vi "DCHX Dehumidification Setup_V17.vi"() -> ()   [LabVIEW 2018]
uses:
  <vilib>/DAQmx/write.llb/DAQmx Write (Analog DBL 1Chan 1Samp).vi
  <vilib>/DAQmx/write.llb/DAQmx Write (Digital Bool 1Line 1Point).vi
  <vilib>/DAQmx/read.llb/DAQmx Read (Analog 1D Wfm NChan 1Samp).vi
  <vilib>/DAQmx/create/channels.llb/DAQmx Create Channel (AI-Temperature-Thermocouple).vi
  <vilib>/DAQmx/create/channels.llb/DAQmx Create Channel (AI-Voltage-Basic).vi
  <vilib>/DAQmx/create/channels.llb/DAQmx Create Channel (DO-Digital Output).vi
  <vilib>/Instr/_visa.llb/VISA Configure Serial Port (Instr).vi
  <vilib>/DAQmx/create/channels.llb/DAQmx Create Channel (AO-Voltage-Basic).vi
  <vilib>/DAQmx/create/channels.llb/DAQmx Create Channel (AI-Current-Basic).vi
  <vilib>/DAQmx/miscellaneous.llb/DAQmx Fill In Error Info.vi
  <vilib>/Waveform/WDTOps.llb/WDT Get XY Value DBL.vi
  <vilib>/Analysis/polynomials.llb/Scalar Polynomial Evaluation (DBL).vi
  <resource>/objmgr/daqmx.rc
  <vilib>/Analysis/NI_AALPro.lvlib
panel:
  in  "Reset":bool
  out "RH2":dbl
  out "RH1":dbl
  out "error out 3":errorcluster
  out "error out 2":errorcluster
  in  "Tab Control 1":enum32{"Controls", "Channels", "Calibration"}(tab)
  in  "Cold Chiller Power":bool
  in  "Cold Chiller Setpoint":dbl=30.0 format="%.3g"
  in  "Hot Chiller Power":bool
  in  "Hot Chiller Setpoint":dbl=30.0 format="%.3g"
  in  "Fan Speed Setpoint (0-10V)":dbl min=0.0 max=10.0
  in  "Start test":bool
  in  "Number of complete cycles":dbl
  out "Number of Half-Cycles":dbl
  in  "Heating time (sec)":dbl=7.0 caption="Time Target (s)"
  in  "Cooling time (sec)":dbl=3.0 caption="Time Target (s)"
  out "Elapsed Half-Cycle Time (s)":dbl format="%#_3g"
  in  "Heating/Cooling Status":bool
  in  "Humidity/Temp Sensors":tag="cDAQ6Mod1/ai0:3"
  in  "Thermocouples":tag="cDAQ6Mod2/ai0:1"
  in  "Solenoid Channel":tag="cDAQ6Mod4/port0/line0"
  in  "Solenoid Channel 2":tag="cDAQ6Mod4/port0/line1"
  in  "Cold Chiller Port":refnum<visa-resource-name>="COM3"
  in  "Hot Chiller Port":refnum<visa-resource-name>="COM3"
  in  "Fans (Output)":tag="cDAQ6Mod3/ao0"
  in  "DUK Flow Meter":tag="cDAQ6Mod1/ai9"
  in  "Differential Pressure Current":tag="cDAQ6Mod1/ai8"
  in  "DUK FLow Meter scale":dbl=1245.0 format="%0.2f"
  in  "DUK FLow Meter offset":dbl=-4.9
  in  "RTD1 offset":dbl=-2.53 format="%0.2f"
  in  "RTD2 offset":dbl=-3.22 format="%0.2f"
  in  "RTD1 scale":dbl=5.6286 format="%0.2f"
  in  "RTD2 scale":dbl=5.701 format="%0.2f"
  in  "RH1 offset":ext=0.1906
  in  "RH2 offset":ext=0.246
  in  "RH1  scale":ext=10.58
  in  "RH2 scale":ext=10.3599999999999999997
  in  "TC-T1 offset":dbl format="%0.2f"
  in  "TC-T1 scale":dbl=1.0 format="%0.2f"
  in  "TC-T2 offset":dbl format="%0.2f"
  in  "TC-T2 scale":dbl=1.0 format="%0.2f"
  in  "Scale DiffP 1":dbl=124945.0 format="%#_13g"
  in  "offset DiffP":dbl=-1504.3 format="%0.2f"
  in  "stop":bool
  in  "Tab Control 2":enum32{"All Data Graphs"}(tab)
  out "Air Flow Rate (CFM)":waveform(dbl)(graph)
  out "DUK Flow Meter":waveform(dbl)(graph)
  out "RTD Temeprature - KIMO":waveform(dbl)[](graph)
  out "Relative Humidity - KIMO":waveform(dbl)[](graph)
  out "Temperature-TC":waveform(dbl)[](graph)
  out "Absolute Humidity Chart":waveform(dbl)[](graph)
  out "Orifice Pressure (Pa)":waveform(dbl)(graph)
  out "Percent Error":dbl
  # "Cooling"
  # "Heating"
  # "Air Side"
  # "Liquid Side"
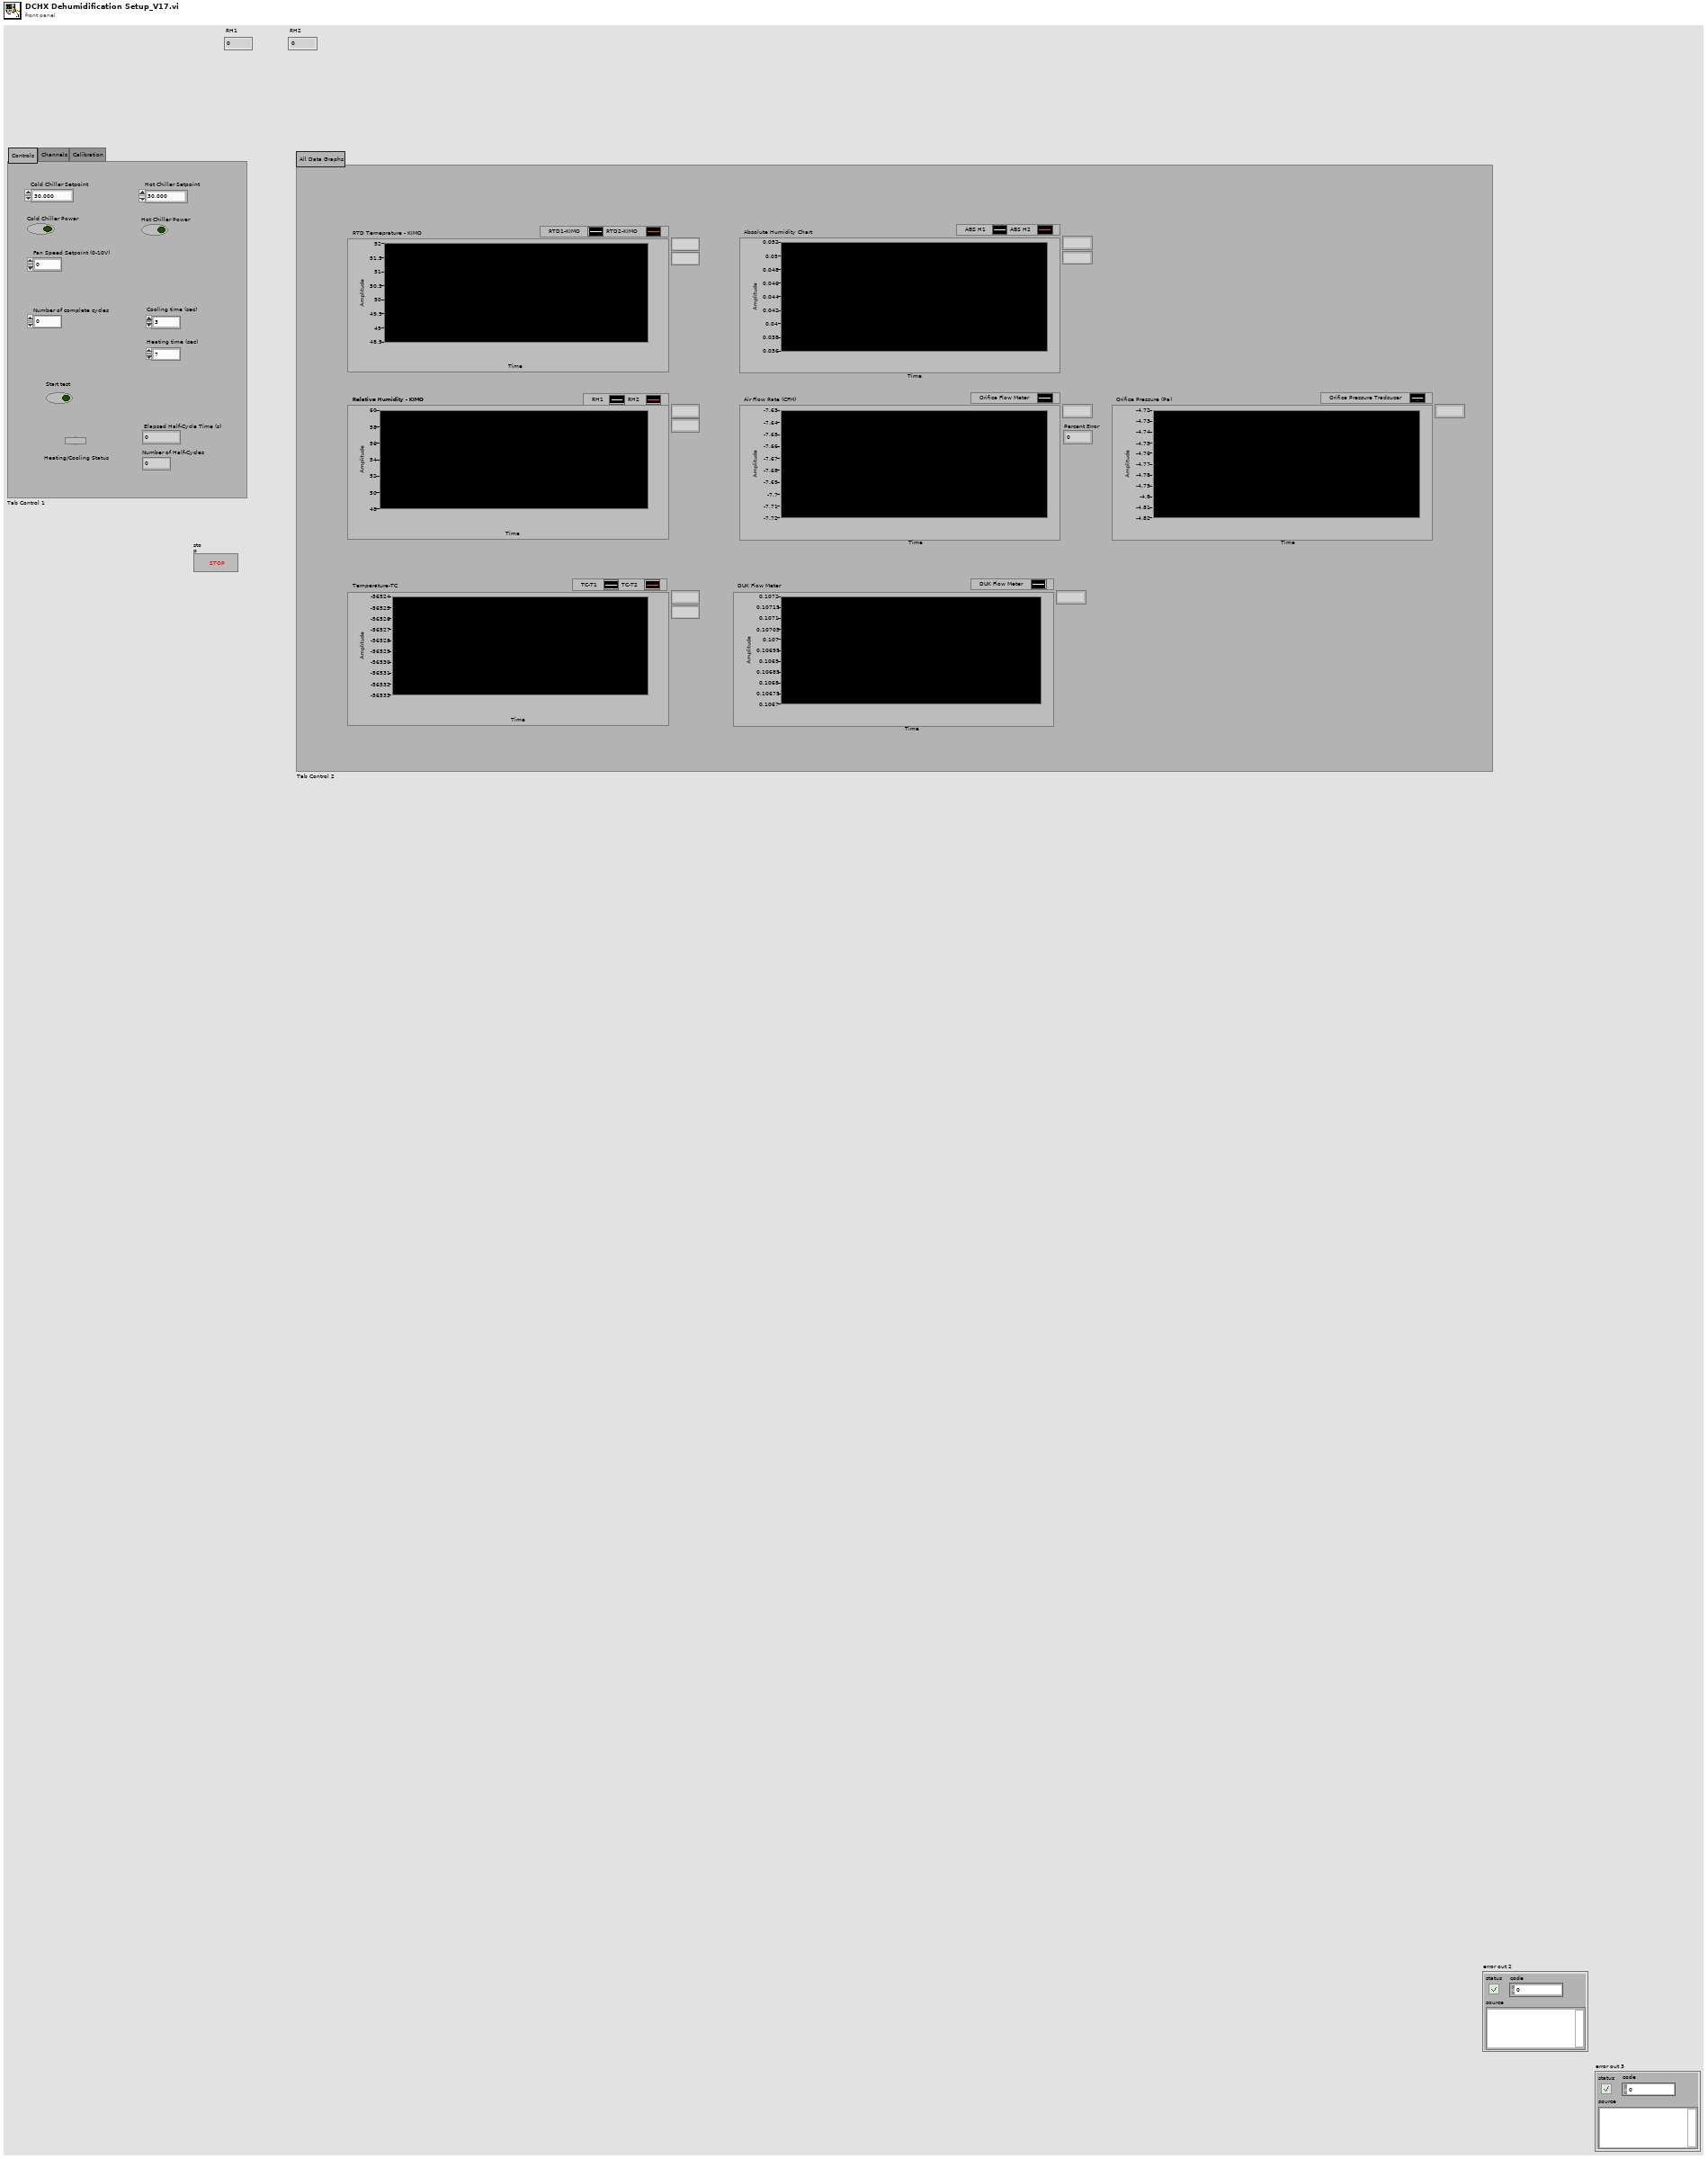
[diagram p1: front panel]
types:
  T1 = enum8{"Enabled", "Disabled", "Disabled and Grayed Out"}
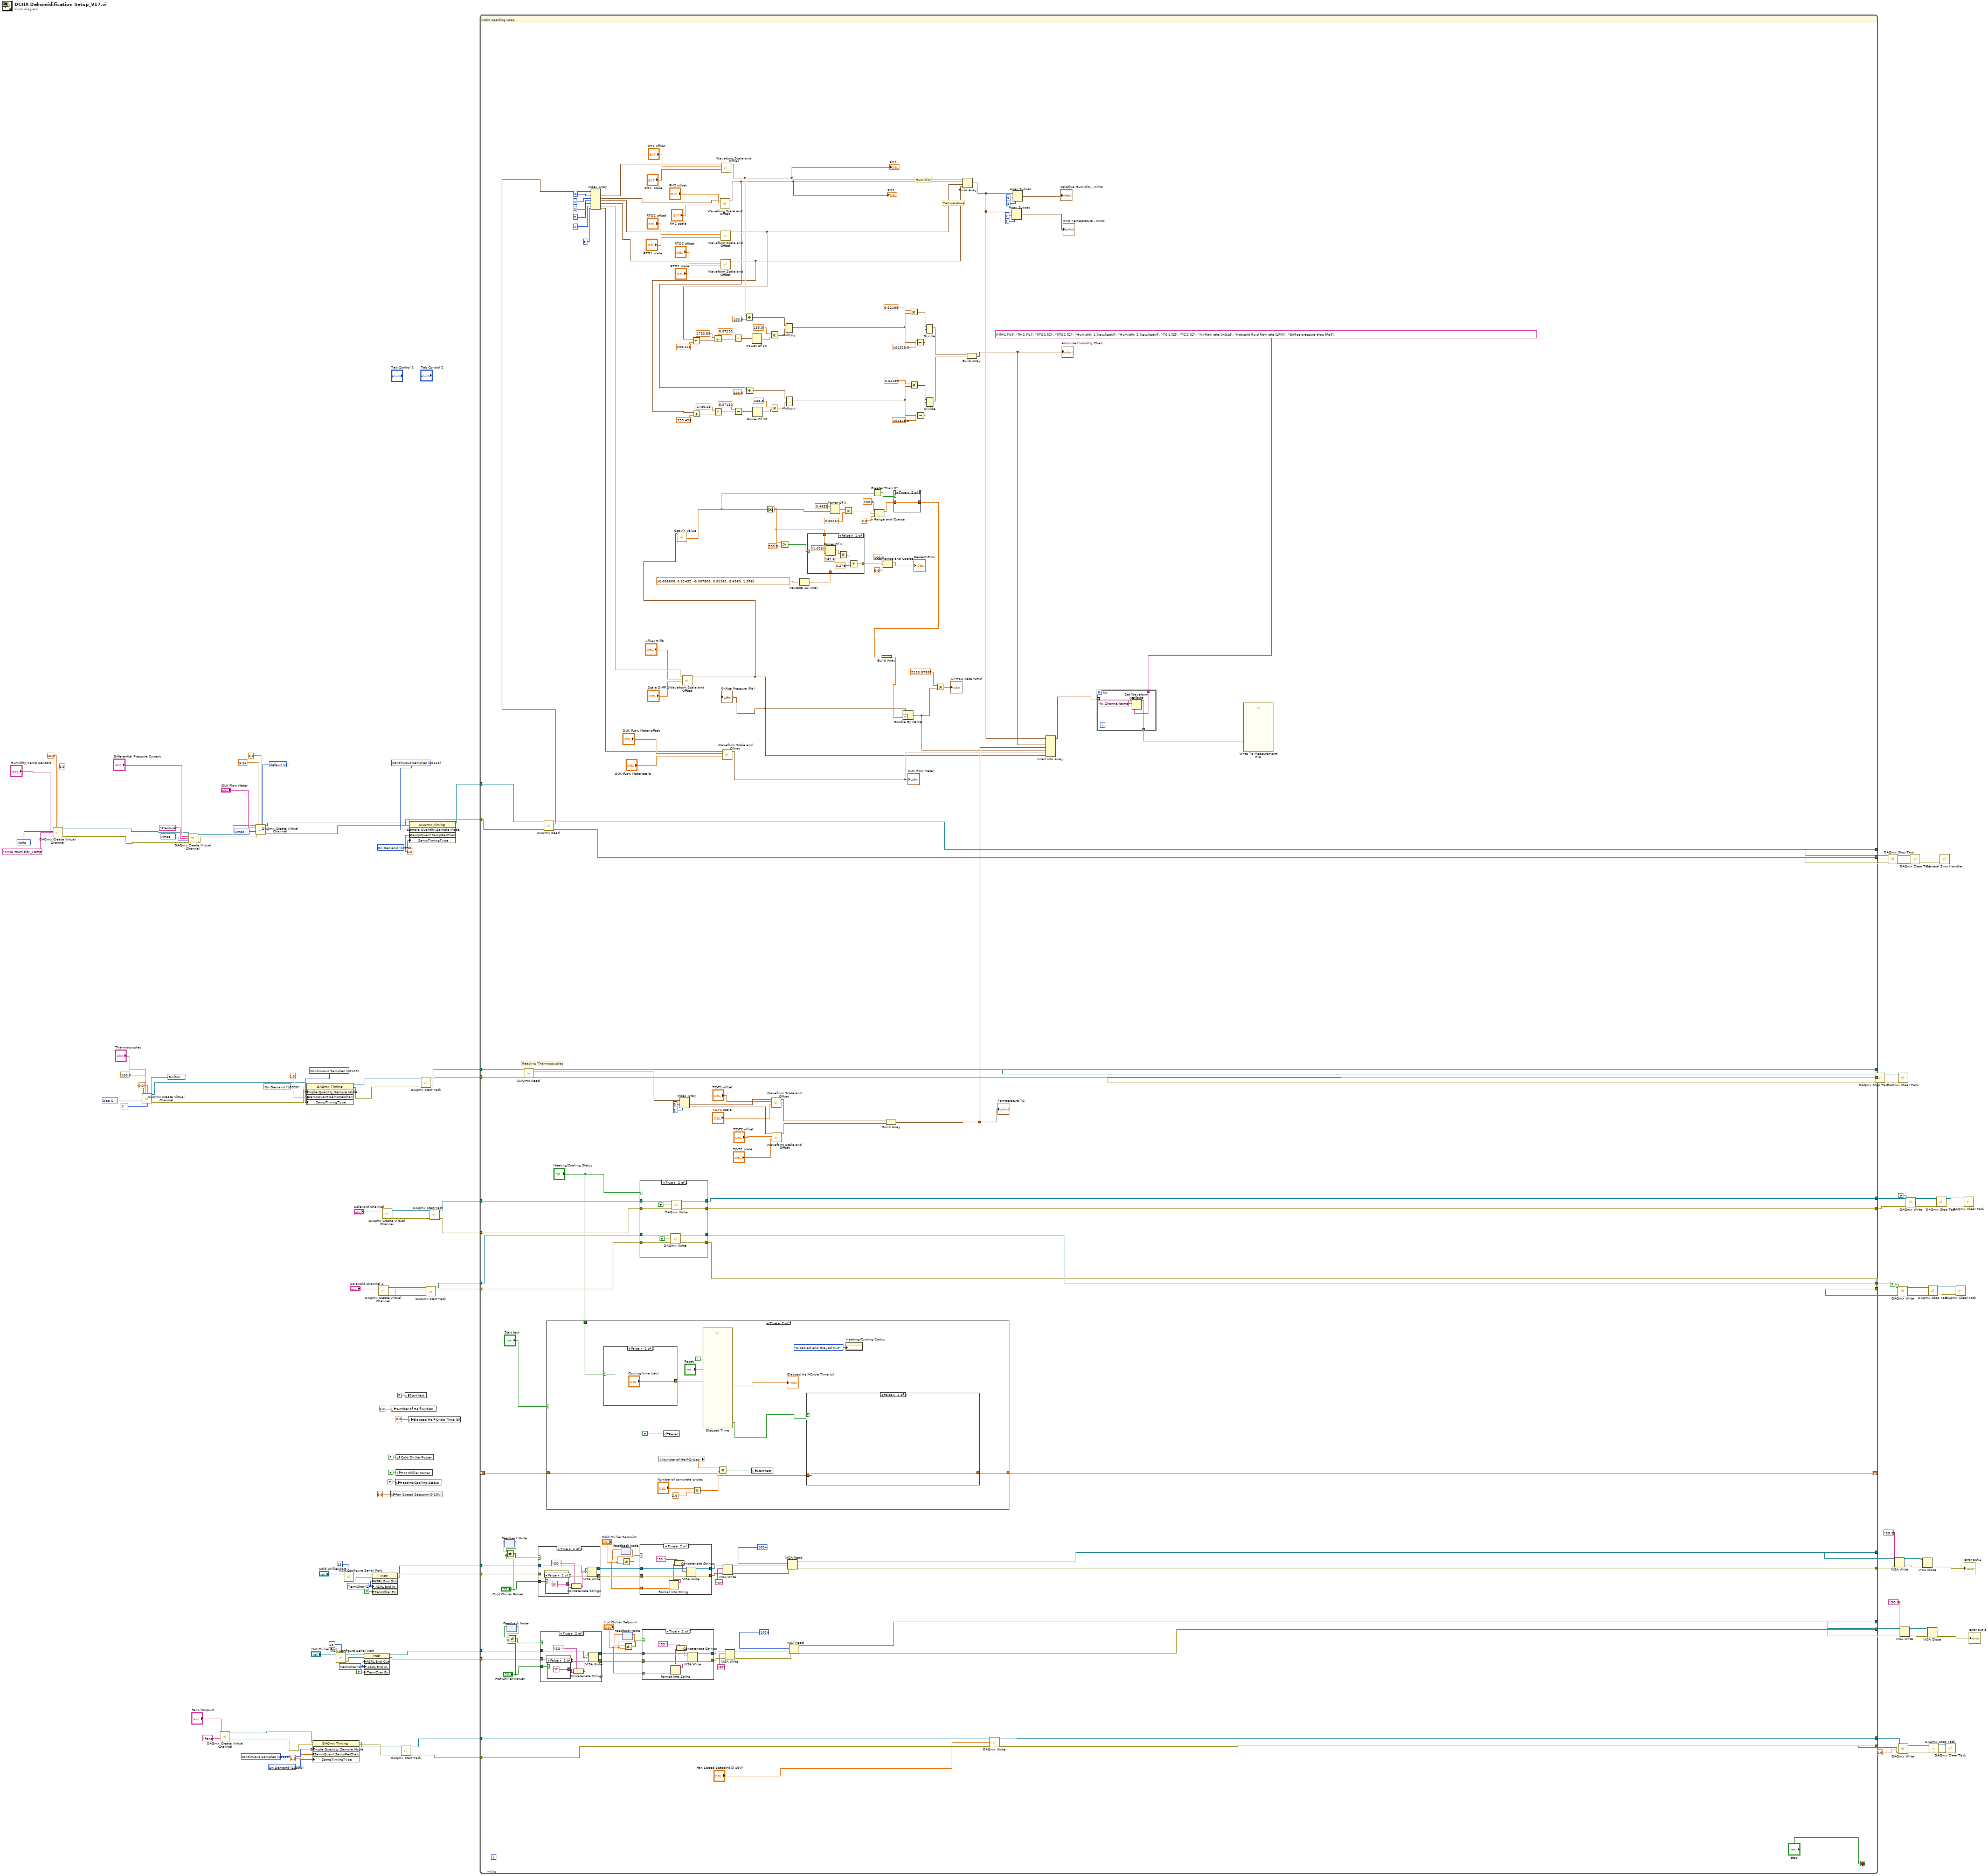
[diagram p0: block diagram]
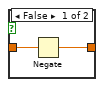
[diagram p2: hidden frame]
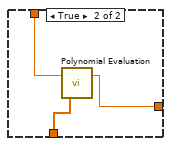
[diagram p3: hidden frame]
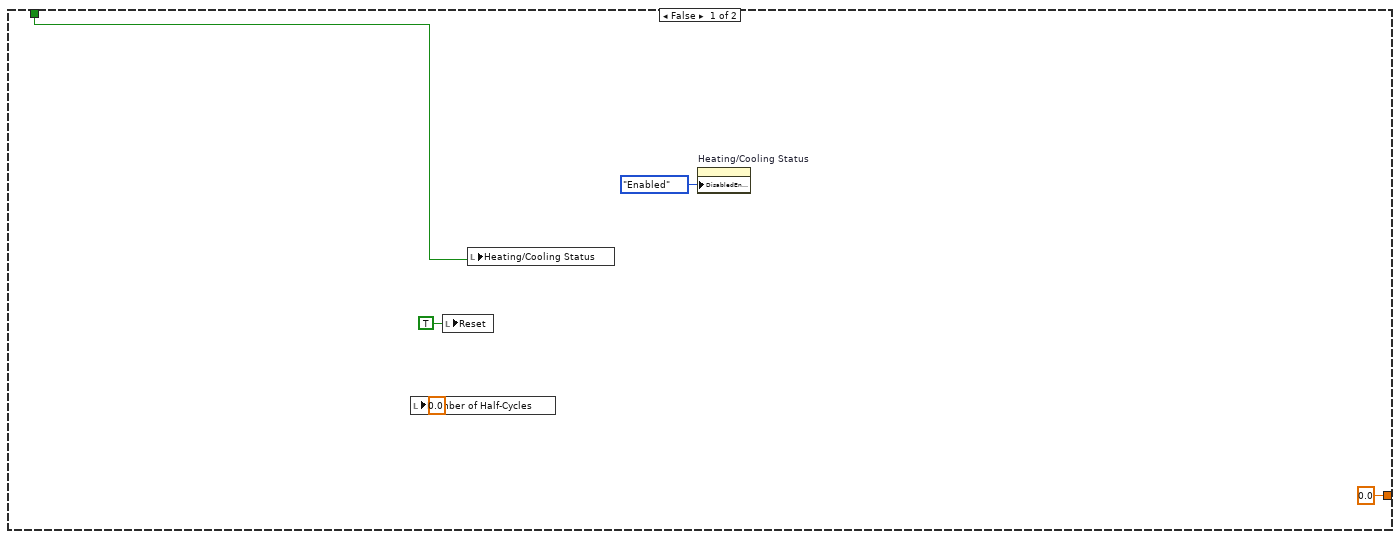
[diagram p4: hidden frame]
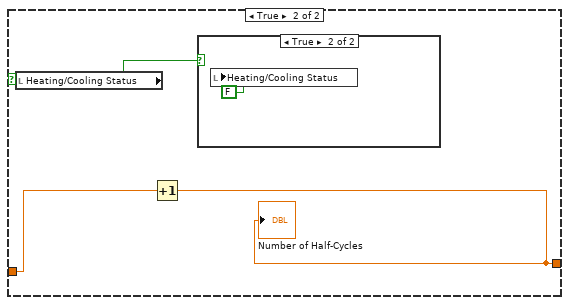
[diagram p5: hidden frame]
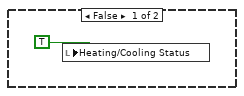
[diagram p6: hidden frame]
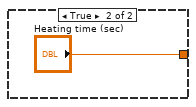
[diagram p7: hidden frame]
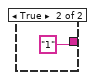
[diagram p10: hidden frame]
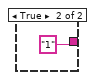
[diagram p13: hidden frame]
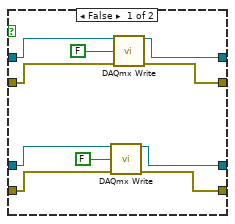
[diagram p14: hidden frame]
diagram:
  w18 = 10342 items=["Amps"=10342, "From Custom Scale"=10065] ("units")
  w23 = -1 items=["default"=-1, "RSE"=10083, "NRSE"=10078, "Differential"=10106, "Pseudodifferential"=12529] ("input terminal configuration")
  w26 = 10342 items=["Amps"=10342, "From Custom Scale"=10065] ("units")
  w38 = 10390 items=["Sample Clock"=10388, "Burst Handshake"=12548, "Handshake"=10389, "Implicit"=10451, "On Demand"=10390, "Change Detection"=12504, "Pipelined Sample Clock"=14668] ("SampTimingType")
  w40 = 10123 items=["Finite Samples"=10178, "Continuous Samples"=10123, "Hardware Timed Single Point"=12522] ("SampQuant.SampMode")
  w49 = u16 2 items=["None", "Last Bit", "TermChar"] ("Serial Settings:End Mode for Reads")
  w63 = u16 2 items=["None", "Last Bit", "TermChar"] ("Serial Settings:End Mode for Reads")
  w104 = 10348 items=["Volts"=10348, "From Custom Scale"=10065] ("units")
  w105 = 10390 items=["Sample Clock"=10388, "Burst Handshake"=12548, "Handshake"=10389, "Implicit"=10451, "On Demand"=10390, "Change Detection"=12504, "Pipelined Sample Clock"=14668] ("SampTimingType")
  w107 = 10123 items=["Finite Samples"=10178, "Continuous Samples"=10123, "Hardware Timed Single Point"=12522] ("SampQuant.SampMode")
  w112 = 10390 items=["Sample Clock"=10388, "Burst Handshake"=12548, "Handshake"=10389, "Implicit"=10451, "On Demand"=10390, "Change Detection"=12504, "Pipelined Sample Clock"=14668] ("SampTimingType")
  w113 = 10123 items=["Finite Samples"=10178, "Continuous Samples"=10123, "Hardware Timed Single Point"=12522] ("SampQuant.SampMode")
  w117 = 10086 items=["J"=10072, "K"=10073, "N"=10077, "R"=10082, "S"=10085, "T"=10086, "B"=10047, "E"=10055] ("thermocouple type")
  w118 = 10200 items=["Built-In"=10200, "Constant Value"=10116, "Channel"=10113] ("cjc source")
  w119 = 10143 items=["Deg C"=10143, "Deg F"=10144, "Kelvins"=10325, "Deg R"=10145, "From Custom Scale"=10065] ("units")
  n1 = call-poly <vilib>:"DAQmx Create Virtual Channel.vi"("maximum value"=10.0, "minimum value"=0.0, "physical channels"="Humidity/Temp Sensors", "name to assign"="KIMO Humidity_Temp", "units"=w104) -> ("task out"=w14:refnum<k21>, "error out"=w15:errorcluster)  [unwired: 9 in]
  n2 = call-poly <vilib>:"DAQmx Create Virtual Channel.vi"("maximum value"=100.0, "minimum value"=0.0, "physical channels"="Thermocouples", "cjc source"=w118, "units"=w119, "thermocouple type"=w117) -> ("task out"=w109:refnum<k21>, "error out"=w108:errorcluster)  [unwired: 8 in]
  n3 = call-poly <vilib>:"DAQmx Create Virtual Channel.vi"("task in"=w14, "physical channels"="Differential Pressure Current", "name to assign"="Pressure", "units"=w18, "error in"=w15) -> ("task out"=w17:refnum<k21>, "error out"=w16:errorcluster)  [unwired: 9 in]
  n4 = call-poly <vilib>:"DAQmx Create Virtual Channel.vi"("physical channels"="Fans (Output)", "name to assign"="Fans") -> ("task out"=w35:refnum<k21>, "error out"=w36:errorcluster)  [unwired: 12 in]
  n5 = call-poly <vilib>:"DAQmx Create Virtual Channel.vi"("task in"=w17, "maximum value"=0.02, "minimum value"=0.0, "input terminal configuration"=w23, "physical channels"="DUK Flow Meter", "units"=w26, "error in"=w16) -> ("task out"=w22:refnum<k21>, "error out"=w21:errorcluster)  [unwired: 7 in]
  n6 = property class="DAQmx Timing"(reference=w109, error in=w108, "Sample Quantity:Sample Mode"=w113, "SampQuant.SampPerChan"=1.0, "SampTimingType"=w112) -> (reference out=w111:refnum<k21>, error out=w110:errorcluster)
  n7 = property class="DAQmx Timing"(reference=w35, error in=w36, "Sample Quantity:Sample Mode"=w40, "SampQuant.SampPerChan"=1.0, "SampTimingType"=w38) -> (reference out=w29:refnum<k21>, error out=w28:errorcluster)
  n8 = call-poly "VISA Configure Serial Port"("VISA resource name"="Hot Chiller Port", "termination char\n(0xA = '\\n' = LF)"=u8 13 ("termination char\n(0xA = '\\n' = LF)")) -> ("VISA resource name out"=w46:refnum<visa-resource-name>, "error out"=w47:errorcluster)  [unwired: 12 in]
  n9 = call-poly "VISA Configure Serial Port"("VISA resource name"="Cold Chiller Port", "termination char\n(0xA = '\\n' = LF)"=u8 13 ("termination char\n(0xA = '\\n' = LF)")) -> ("VISA resource name out"=w60:refnum<visa-resource-name>, "error out"=w61:errorcluster)  [unwired: 12 in]
  n10 = property class="Instr"(reference=w46, error in=w47, "ASRL End Out"=w49, "ASRL End In"=w49, "TermChar En"=FALSE ("Message Based Settings:Termination Character Enable")) -> (reference out=w44:refnum<visa-resource-name>, error out=w43:errorcluster)
  n11 = property class="Instr"(reference=w60, error in=w61, "ASRL End Out"=w63, "ASRL End In"=w63, "TermChar En"=FALSE ("Message Based Settings:Termination Character Enable")) -> (reference out=w58:refnum<visa-resource-name>, error out=w57:errorcluster)
  n12 = call-poly <vilib>:"DAQmx Create Virtual Channel.vi"("lines"="Solenoid Channel 2") -> ("task out"=w78:refnum<k21>, "error out"=w79:errorcluster)  [unwired: 13 in]
  n13 = call-poly <vilib>:"DAQmx Create Virtual Channel.vi"("lines"="Solenoid Channel") -> ("task out"=w90:refnum<k21>, "error out"=w91:errorcluster)  [unwired: 13 in]
  n14 = local write "Fan Speed Setpoint (0-10V)"(0.0 ("Fan Speed Setpoint (0-3600 RPM)")) -> ()
  n15 = local write "Number of Half-Cycles"(0.0 ("Cycles")) -> ()
  n16 = local write "Heating/Cooling Status"(FALSE ("Heating/Cooling Status")) -> ()
  n17 = local write "Cold Chiller Power"(FALSE ("Cold Chiller Power")) -> ()
  n18 = local write "Hot Chiller Power"(FALSE ("Hot Chiller Power")) -> ()
  n19 = call <vilib>:"DAQmx Start Task.vi"("task/channels in"=w29, "error in"=w28) -> ("task out"=w31:refnum<k21>, "error out"=w30:errorcluster)  [unwired: 12 in]
  n20 = local write "Start test"(FALSE ("Start test")) -> ()
  n21 = local write "Elapsed Half-Cycle Time (s)"(0.0 ("Elapsed Time (s)")) -> ()
  n22 = property class="DAQmx Timing"(reference=w22, error in=w21, "Sample Quantity:Sample Mode"=w107, "SampQuant.SampPerChan"=1.0, "SampTimingType"=w105) -> (reference out=w102:refnum<k21>, error out=w101:errorcluster)
  n23 = call <vilib>:"DAQmx Start Task.vi"("task/channels in"=w111, "error in"=w110) -> ("task out"=w121:refnum<k21>, "error out"=w120:errorcluster)  [unwired: 12 in]
  n24 = call <vilib>:"DAQmx Start Task.vi"("task/channels in"=w78, "error in"=w79) -> ("task out"=w76:refnum<k21>, "error out"=w13:errorcluster)  [unwired: 12 in]
  n25 = call <vilib>:"DAQmx Start Task.vi"("task/channels in"=w90, "error in"=w91) -> ("task out"=w83:refnum<k21>, "error out"=w82:errorcluster)  [unwired: 12 in]
  n26 = while {
    tunnel: w121 -> [w298]
    tunnel: w120 -> [w297]
    tunnel: [w296] -> w125
    tunnel: [w295] -> w123
    tunnel: w102 -> [w294]
    tunnel: w101 -> [w293]
    tunnel: [w292] -> w97
    tunnel: [w291] -> w96
    tunnel: w83 -> [w253]
    tunnel: w82 -> [w252]
    tunnel: [w251] -> w81
    tunnel: [w250] -> w80
    tunnel: w76 -> [w249]
    tunnel: [w248] -> w70
    tunnel: [w247] -> w69
    tunnel: w58 -> [w232]
    tunnel: w57 -> [w231]
    tunnel: [w230] -> w56
    tunnel: [w229] -> w55
    tunnel: w44 -> [w214]
    tunnel: w43 -> [w213]
    tunnel: [w212] -> w42
    tunnel: [w211] -> w41
    tunnel: [w210] -> w5
    tunnel: [w209] -> w4
    tunnel: w31 -> [w208]
    tunnel: w30 -> [w207]
    tunnel: w13 -> [w159]
    shift-right: [w153] -> _
    shift-left: _ -> [w154]
    stop <- "stop" stop-if-true
    # "Temperature"
    # "Humidity"
    # "Reading Thermocouples"
    # "Main Reading Loop"
    n27 = feedback #1() -> (w240:bool)  [unwired: 1 in]
    n28 = feedback-in #1("Cold Chiller Power") -> ()
    n29 = Not Equal?(x=w240, y="Cold Chiller Power") -> (x != y?=w238:bool)
    n30 = feedback #2() -> (w222:bool)  [unwired: 1 in]
    n31 = feedback-in #2("Hot Chiller Power") -> ()
    n32 = Not Equal?(x=w222, y="Hot Chiller Power") -> (x != y?=w220:bool)
    n33 = call-poly <vilib>:"DAQmx Read.vi"("task/channels in"=w298, "error in"=w297) -> ("task out"=w296:refnum<k21>, "data"=w274:waveform(dbl)[], "error out"=w295:errorcluster)  [unwired: 11 in]
    n34 = case shown="True" w238 {
      tunnel: w232 -> [w377 w382]
      tunnel: w231 -> [w376 w381]
      tunnel: [w377 w380] -> w242
      tunnel: [w376 w379] -> w241
      tunnel: "Cold Chiller Power" -> [_ w378]
      frame False {
      }
      frame True {
        n35 = case shown="False" w378 {
          tunnel: ["0" ("write buffer") "1" ("write buffer")] -> w383
          frame False {
          }
          frame True {
          }
        }
        n36 = Concatenate Strings("SO " ("write buffer"), w383) -> (w384:string)
        n37 = VISA Write(VISA resource name=w382, write buffer=w384, error in (no error)=w381) -> (VISA resource name out=w380:refnum<visa-resource-name>, error out=w379:errorcluster)  [unwired: 1 out]
      }
    }
    n38 = case shown="True" w220 {
      tunnel: w214 -> [w355 w360]
      tunnel: w213 -> [w354 w359]
      tunnel: [w355 w358] -> w224
      tunnel: [w354 w357] -> w223
      tunnel: "Hot Chiller Power" -> [_ w356]
      frame False {
      }
      frame True {
        n39 = case shown="False" w356 {
          tunnel: ["0" ("write buffer") "1" ("write buffer")] -> w361
          frame False {
          }
          frame True {
          }
        }
        n40 = Concatenate Strings("SO " ("write buffer"), w361) -> (w362:string)
        n41 = VISA Write(VISA resource name=w360, write buffer=w362, error in (no error)=w359) -> (VISA resource name out=w358:refnum<visa-resource-name>, error out=w357:errorcluster)  [unwired: 1 out]
      }
    }
    n42 = call-poly <vilib>:"DAQmx Read.vi"("task/channels in"=w294, "error in"=w293) -> ("task out"=w292:refnum<k21>, "data"=w290:waveform(dbl)[], "error out"=w291:errorcluster)  [unwired: 11 in]
    n43 = case shown="True" "Start test" {
      tunnel: "Heating/Cooling Status" -> [w317 w330]
      tunnel: w154 -> [_ w323]
      tunnel: [0.0 w322] -> w153
      frame False {
        n44 = local write "Number of Half-Cycles"(0.0 ("Cycles")) -> ()
        n45 = local write "Reset"(TRUE ("Reset")) -> ()
        n46 = local write "Heating/Cooling Status"(w317) -> ()
        n47 = property on="Heating/Cooling Status" class="Bool (strict)"("DisabledEnum"=T1."Enabled" ("Disabled")) -> ()  [unwired: 2 in, 2 out]
      }
      frame True {
        n48 = case shown="False" w330 {
          tunnel: ["Cooling time (sec)" "Heating time (sec)"] -> w329
          frame False {
          }
          frame True {
          }
        }
        n49 = local read "Number of Half-Cycles"() -> (w328:dbl)
        n50 = local write "Reset"(FALSE ("Reset")) -> ()
        n51 = Multiply(x="Number of complete cycles", y=2.0) -> (x*y=w327:dbl)
        n52 = call "Elapsed Time"("Time Target (s)"=w329, "Reset"="Reset", "Auto Reset"=TRUE) -> ("Elapsed Time (s)"=→"Elapsed Half-Cycle Time (s)":dbl, "Time has Elapsed"=w334:bool)  [unwired: 9 in, 6 out]
        n53 = Less?(x=w328, y=w327) -> (x < y?=w324:bool)
        n54 = local write "Start test"(w324) -> ()
        n55 = case shown="False" w334 {
          tunnel: w323 -> [w336 w338]
          tunnel: [w336 w337] -> w322
          frame False {
          }
          frame True {
            n56 = local read "Heating/Cooling Status"() -> (w339:bool)
            n57 = Increment(x=w338) -> (x+1=w337:dbl)
            "Number of Half-Cycles" <- w337
            n58 = case shown="True" w339 {
              frame False {
                n59 = local write "Heating/Cooling Status"(TRUE ("Status")) -> ()
              }
              frame True {
                n60 = local write "Heating/Cooling Status"(FALSE ("Status")) -> ()
              }
            }
          }
        }
        n61 = property on="Heating/Cooling Status" class="Bool (strict)"("DisabledEnum"=T1."Disabled and Grayed Out" ("Disabled")) -> ()  [unwired: 2 in, 2 out]
      }
    }
    n62 = Index Array(array=w290, index #1=0 ("index"), index #2=1 ("index"), index #3=2 ("index"), index #4=3 ("index"), index #5=4 ("index"), index #6=5 ("index")) -> (element #1=w280:waveform(dbl), element #2=w279:waveform(dbl), element #3=w278:waveform(dbl), element #4=w277:waveform(dbl), element #5=w163:waveform(dbl), element #6=w162:waveform(dbl))
    n63 = feedback #3() -> (w237:dbl)  [unwired: 1 in]
    n64 = feedback-in #3("Cold Chiller Setpoint") -> ()
    n65 = Not Equal?(x=w237, y="Cold Chiller Setpoint") -> (x != y?=w236:bool)
    n66 = feedback #4() -> (w219:dbl)  [unwired: 1 in]
    n67 = feedback-in #4("Hot Chiller Setpoint") -> ()
    n68 = Not Equal?(x=w219, y="Hot Chiller Setpoint") -> (x != y?=w218:bool)
    n69 = case shown="True" "Heating/Cooling Status" {
      tunnel: w253 -> [w395 w407]
      tunnel: w252 -> [w392 w406]
      tunnel: [w393 w405] -> w250
      tunnel: [w394 w404] -> w251
      tunnel: w249 -> [w391 w403]
      tunnel: w159 -> [w390 w402]
      tunnel: [w389 w401] -> w248
      tunnel: [w388 w400] -> w247
      frame False {
        n70 = call-poly <vilib>:"DAQmx Write.vi"("task/channels in"=w391, "data"=FALSE, "error in"=w390) -> ("task out"=w389:refnum<k21>, "error out"=w388:errorcluster)  [unwired: 10 in, 1 out]
        n71 = call-poly <vilib>:"DAQmx Write.vi"("task/channels in"=w395, "data"=FALSE, "error in"=w392) -> ("task out"=w394:refnum<k21>, "error out"=w393:errorcluster)  [unwired: 10 in, 1 out]
      }
      frame True {
        n72 = call-poly <vilib>:"DAQmx Write.vi"("task/channels in"=w403, "data"=TRUE, "error in"=w402) -> ("task out"=w401:refnum<k21>, "error out"=w400:errorcluster)  [unwired: 10 in, 1 out]
        n73 = call-poly <vilib>:"DAQmx Write.vi"("task/channels in"=w407, "data"=TRUE, "error in"=w406) -> ("task out"=w404:refnum<k21>, "error out"=w405:errorcluster)  [unwired: 10 in, 1 out]
      }
    }
    n74 = case shown="True" w236 {
      tunnel: w242 -> [w367 w375]
      tunnel: w241 -> [w366 w374]
      tunnel: [w367 w372] -> w234
      tunnel: [w366 w373] -> w233
      tunnel: "Cold Chiller Setpoint" -> [_ w368]
      frame False {
      }
      frame True {
        n75 = Format Into String(w368) -> (resulting string=w369:string)  [unwired: 3 in, 1 out]
        n76 = Concatenate Strings("SS " ("write buffer"), w369) -> (w370:string)
        n77 = VISA Write(VISA resource name=w375, write buffer=w370, error in (no error)=w374) -> (VISA resource name out=w372:refnum<visa-resource-name>, error out=w373:errorcluster)  [unwired: 1 out]
      }
    }
    n78 = case shown="True" w218 {
      tunnel: w224 -> [w345 w353]
      tunnel: w223 -> [w344 w352]
      tunnel: [w345 w350] -> w216
      tunnel: [w344 w351] -> w215
      tunnel: "Hot Chiller Setpoint" -> [_ w346]
      frame False {
      }
      frame True {
        n79 = Format Into String(w346) -> (resulting string=w347:string)  [unwired: 3 in, 1 out]
        n80 = Concatenate Strings("SS " ("write buffer"), w347) -> (w348:string)
        n81 = VISA Write(VISA resource name=w353, write buffer=w348, error in (no error)=w352) -> (VISA resource name out=w350:refnum<visa-resource-name>, error out=w351:errorcluster)  [unwired: 1 out]
      }
    }
    n82 = Index Array(array=w274, index #1=0 ("index"), index #2=1 ("index")) -> (element #1=w271:waveform(dbl), element #2=w270:waveform(dbl))
    n83 = call <vilib>:"Waveform Scale and Offset.vi"("scale"="Scale DiffP 1", "offset"="offset DiffP", "waveform in"=w163) -> ("waveform out"=w130:waveform(dbl))  [unwired: 7 in, 1 out]
    "Orifice Pressure (Pa)" <- w130
    n84 = call-poly <vilib>:"Get XY Value.vi"("waveform in"=w130) -> ("Y value"=w129:dbl)  [unwired: 6 in, 4 out]
    n85 = call <vilib>:"Waveform Scale and Offset.vi"("scale"="RH2 scale", "offset"="RH2 offset", "waveform in"=w279) -> ("waveform out"=w168:waveform(dbl))  [unwired: 7 in, 1 out]
    "RH2" <- w168
    n86 = call <vilib>:"Waveform Scale and Offset.vi"("scale"="RTD1 scale", "offset"="RTD1 offset", "waveform in"=w278) -> ("waveform out"=w170:waveform(dbl))  [unwired: 7 in, 1 out]
    n87 = Add(x=w170, y=233.426) -> (x+y=w204:waveform(dbl))
    n88 = Divide(x=1730.63, y=w204) -> (x/y=w202:waveform(dbl))
    n89 = call <vilib>:"Waveform Scale and Offset.vi"("scale"="RTD2 scale", "offset"="RTD2 offset", "waveform in"=w277) -> ("waveform out"=w169:waveform(dbl))  [unwired: 7 in, 1 out]
    n90 = Add(x=w169, y=233.426) -> (x+y=w188:waveform(dbl))
    n91 = Divide(x=1730.63, y=w188) -> (x/y=w186:waveform(dbl))
    n92 = call <vilib>:"Waveform Scale and Offset.vi"("scale"="RH1  scale", "offset"="RH1 offset", "waveform in"=w280) -> ("waveform out"=w171:waveform(dbl))  [unwired: 7 in, 1 out]
    "RH1" <- w171
    n93 = call <vilib>:"Waveform Scale and Offset.vi"("scale"="DUK FLow Meter scale", "offset"="DUK FLow Meter offset", "waveform in"=w162) -> ("waveform out"=w160:waveform(dbl))  [unwired: 7 in, 1 out]
    "DUK Flow Meter" <- w160
    n94 = VISA Write(VISA resource name=w234, write buffer="RT", error in (no error)=w233) -> (VISA resource name out=w245:refnum<visa-resource-name>, error out=w244:errorcluster)  [unwired: 1 out]
    n95 = VISA Write(VISA resource name=w216, write buffer="RT", error in (no error)=w215) -> (VISA resource name out=w227:refnum<visa-resource-name>, error out=w226:errorcluster)  [unwired: 1 out]
    n96 = Subtract(x=8.07131, y=w202) -> (x-y=w200:waveform(dbl))
    n97 = Subtract(x=8.07131, y=w186) -> (x-y=w184:waveform(dbl))
    n98 = Divide(x=w171, y=100.0) -> (x/y=w192:waveform(dbl))
    n99 = Divide(x=w168, y=100.0) -> (x/y=w176:waveform(dbl))
    n100 = Power Of 10(x=w200) -> (10^x=w199:waveform(dbl))
    n101 = Power Of 10(x=w184) -> (10^x=w183:waveform(dbl))
    n102 = Absolute Value(x=w129) -> (abs(x)=w137:dbl)
    n103 = Multiply(x=133.3, y=w199) -> (x*y=w197:waveform(dbl))
    n104 = Multiply(x=133.3, y=w183) -> (x*y=w181:waveform(dbl))
    n105 = call <vilib>:"Waveform Scale and Offset.vi"("scale"="TC-T1 scale", "offset"="TC-T1 offset", "waveform in"=w271) -> ("waveform out"=w269:waveform(dbl))  [unwired: 7 in, 1 out]
    n106 = call <vilib>:"Waveform Scale and Offset.vi"("scale"="TC-T2 scale", "offset"="TC-T2 offset", "waveform in"=w270) -> ("waveform out"=w268:waveform(dbl))  [unwired: 7 in, 1 out]
    n107 = Greater?(x=w137, y=200.0) -> (0:w145:bool)
    n108 = Multiply(1:w197, 2:w192) -> (0:w190:waveform(dbl))  [unwired: 1 in, 1 out]
    n109 = Multiply(1:w181, 2:w176) -> (0:w174:waveform(dbl))  [unwired: 1 in, 1 out]
    n110 = VISA Read(VISA resource name=w245, byte count=u32 1024, error in (no error)=w244) -> (VISA resource name out=w230:refnum<visa-resource-name>, error out=w229:errorcluster)  [unwired: 2 out]
    n111 = VISA Read(VISA resource name=w227, byte count=u32 1024, error in (no error)=w226) -> (VISA resource name out=w212:refnum<visa-resource-name>, error out=w211:errorcluster)  [unwired: 2 out]
    n112 = Reverse 1D Array(array=dbl[] [-0.006608, 0.01452, -0.007802, 0.01961, 0.4969, 1.586] ("P(x)")) -> (reversed array=w134:dbl[])
    n113 = case shown="False" w145 {
      tunnel: w137 -> [w308 w310]
      tunnel: [w302 w309] -> w141
      tunnel: w134 -> [_ w311]
      frame False {
        n114 = Power Of X(1:w308, 2:-1.026 ("y")) -> (0:w306:dbl)
        n115 = Multiply(x=w306, y=161.6) -> (x*y=w303:dbl)
        n116 = Add(x=w303, y=0.278) -> (x+y=w302:dbl)
      }
      frame True {
        n117 = call-poly <vilib>:"Polynomial Evaluation.vi"("P(x)"=w311, "a"=w310) -> ("P(a)"=w309:dbl)  [unwired: 1 out]
      }
    }
    n118 = Power Of X(1:w137, 2:0.4955 ("y")) -> (0:w148:dbl)
    n119 = Multiply(x=w148, y=0.00167) -> (x*y=w144:dbl)
    n120 = Greater Than 0?(x=w129) -> (x > 0?=w135:bool)
    n121 = In Range and Coerce(upper limit=100.0, x=w144, lower limit=0.0) -> (coerced(x)=w136:dbl)  [unwired: 1 out]
    n122 = In Range and Coerce(upper limit=100.0, x=w141, lower limit=0.0) -> (coerced(x)=→"Percent Error":dbl)  [unwired: 1 out]
    n123 = Build Array(w269, w268) -> (w167:waveform(dbl)[])
    "Temperature-TC" <- w167
    n124 = case shown="True" w135 {
      tunnel: w136 -> [w300 w301]
      tunnel: [w299 w301] -> w131
      frame False {
        n125 = Negate(x=w300) -> (-x=w299:dbl)
      }
      frame True {
      }
    }
    n126 = Build Array(w131) -> (w132:dbl[])
    n127 = Bundle By Name(cluster=w130, "Y"=w132) -> (w128:waveform(dbl))
    n128 = Multiply(x=0.62198, y=w190) -> (x*y=w195:waveform(dbl))
    n129 = Multiply(x=0.62198, y=w174) -> (x*y=w179:waveform(dbl))
    n130 = Subtract(x=101325.0, y=w190) -> (x-y=w194:waveform(dbl))
    n131 = Subtract(x=101325.0, y=w174) -> (x-y=w178:waveform(dbl))
    n132 = Divide(1:w194, 2:w195) -> (0:w173:waveform(dbl))  [unwired: 1 in, 1 out]
    n133 = Divide(1:w178, 2:w179) -> (0:w172:waveform(dbl))  [unwired: 1 in, 1 out]
    n134 = Multiply(x=2118.87997, y=w128) -> (x*y=→"Air Flow Rate (CFM)":waveform(dbl))
    n135 = Build Array(w171, w168, w170, w169) -> (w281:waveform(dbl)[])
    n136 = Build Array(w173, w172) -> (w166:waveform(dbl)[])
    "Absolute Humidity Chart" <- w166
    n137 = call-poly <vilib>:"DAQmx Write.vi"("task/channels in"=w208, "data"="Fan Speed Setpoint (0-10V)", "error in"=w207) -> ("task out"=w210:refnum<k21>, "error out"=w209:errorcluster)  [unwired: 10 in, 1 out]
    n138 = Array Subset(array=w281, index=2, length=2) -> (→"RTD Temeprature - KIMO":waveform(dbl)[])
    n139 = Array Subset(array=w281, index=0, length=2) -> (→"Relative Humidity - KIMO":waveform(dbl)[])
    n140 = Insert Into Array(array=w281, new element #1=w166, new element #2=w167, new element #3=w128, new element #4=w160, new element #5=w130) -> (w150:waveform(dbl)[])  [unwired: 1 in]
    n141 = for {
      tunnel: string[] ["RH1 [%]", "RH2 [%]", "RTD1 [C]", "RTD2 [C]", "Humidity 1 [kgw/kgair]", "Humidity 2 [kgw/kgair]", "TC-1 [C]", "TC-2 [C]", "Air flow rate [m3/s]", "Hot/cold fluid flow rate [LPM]", "Orifice pressure drop [Pa]"] ("Array 3") -> [w315] mode=indexing
      tunnel: w150 -> [w313] mode=indexing
      tunnel: [w312] -> w151 mode=indexing
      n142 = Set Waveform Attribute(5:w315, 6:"NI_ChannelName" ("name"), 7:w313) -> (3:w312:waveform(dbl))  [unwired: 1 in, 2 out]
    }
    n143 = call "Write To Measurement File"("Signals"=w151) -> ()  [unwired: 16 in, 3 out]
  }
  n144 = call <vilib>:"DAQmx Stop Task.vi"("task/channels in"=w125, "error in"=w123) -> ("task out"=w124:refnum<k21>, "error out"=w122:errorcluster)  [unwired: 12 in]
  n145 = call <vilib>:"DAQmx Stop Task.vi"("task/channels in"=w97, "error in"=w96) -> ("task out"=w100:refnum<k21>, "error out"=w99:errorcluster)  [unwired: 12 in]
  n146 = VISA Write(VISA resource name=w56, write buffer="SO 0", error in (no error)=w55) -> (VISA resource name out=w65:refnum<visa-resource-name>, error out=w66:errorcluster)  [unwired: 1 out]
  n147 = call-poly <vilib>:"DAQmx Write.vi"("task/channels in"=w70, "data"=FALSE, "error in"=w69) -> ("task out"=w72:refnum<k21>, "error out"=w71:errorcluster)  [unwired: 10 in, 1 out]
  n148 = call <vilib>:"DAQmx Clear Task.vi"("task in"=w124, "error in"=w122) -> ()  [unwired: 13 in, 1 out]
  n149 = call-poly <vilib>:"DAQmx Write.vi"("task/channels in"=w5, "data"=0.0, "error in"=w4) -> ("task out"=w3:refnum<k21>, "error out"=w2:errorcluster)  [unwired: 10 in, 1 out]
  n150 = VISA Write(VISA resource name=w42, write buffer="SO 0", error in (no error)=w41) -> (VISA resource name out=w51:refnum<visa-resource-name>, error out=w52:errorcluster)  [unwired: 1 out]
  n151 = call-poly <vilib>:"DAQmx Write.vi"("task/channels in"=w81, "data"=FALSE, "error in"=w80) -> ("task out"=w85:refnum<k21>, "error out"=w84:errorcluster)  [unwired: 10 in, 1 out]
  n152 = call <vilib>:"DAQmx Clear Task.vi"("task in"=w100, "error in"=w99) -> ("error out"=w98:errorcluster)  [unwired: 13 in]
  n153 = VISA Close(VISA resource name=w65, error in (no error)=w66) -> (error out=→"error out 2":errorcluster)
  n154 = VISA Close(VISA resource name=w51, error in (no error)=w52) -> (error out=→"error out 3":errorcluster)
  n155 = call <vilib>:"DAQmx Stop Task.vi"("task/channels in"=w72, "error in"=w71) -> ("task out"=w75:refnum<k21>, "error out"=w74:errorcluster)  [unwired: 12 in]
  n156 = call <vilib>:"DAQmx Stop Task.vi"("task/channels in"=w3, "error in"=w2) -> ("task out"=w33:refnum<k21>, "error out"=w32:errorcluster)  [unwired: 12 in]
  n157 = call <vilib>:"DAQmx Stop Task.vi"("task/channels in"=w85, "error in"=w84) -> ("task out"=w88:refnum<k21>, "error out"=w87:errorcluster)  [unwired: 12 in]
  n158 = call <vilib>:"General Error Handler.vi"("error in (no error)"=w98) -> ()  [unwired: 10 in, 5 out]
  n159 = call <vilib>:"DAQmx Clear Task.vi"("task in"=w33, "error in"=w32) -> ()  [unwired: 13 in, 1 out]
  n160 = call <vilib>:"DAQmx Clear Task.vi"("task in"=w75, "error in"=w74) -> ()  [unwired: 13 in, 1 out]
  n161 = call <vilib>:"DAQmx Clear Task.vi"("task in"=w88, "error in"=w87) -> ()  [unwired: 13 in, 1 out]
